vi "Test Get Objects in Range.vi"(11 "Test Case In":refnum<class "Test Object Dictionary.lvclass">) -> (0 "error out":errorcluster, 3 "Test Case Out":refnum<class "Test Object Dictionary.lvclass">)   [LabVIEW 2020, in "Test Object Dictionary.lvclass"]
uses:
  Test Object Dictionary.lvclass
  C:/Program Files/National Instruments/LabVIEW 2026/vi.lib/Astemes/LUnit/Test Case.lvclass
  EDS-File-Viewer/source/Electronic Datasheet/Electronic Datasheet.lvclass/Electronic Datasheet.ctl
  source/Object Entry/Object Entry.lvclass/Object Entry.ctl
  source/Sub Object/Sub Object.lvclass/Sub Object.ctl
  <vilib>/Astemes/LUnit/Test Case.lvclass/Test Case.ctl
  source/Sub Object/Sub Object.lvclass
  EDS-File-Viewer/source/Electronic Datasheet/Electronic Datasheet.lvclass
  source/Typedefs/Object Type.ctl
  source/CANopen.lvlib
  <vilib>/Astemes/LUnit/Test Case.lvclass
  source/Object Dictionary/Object Dictionary.lvclass
  source/Object Entry/Object Entry.lvclass
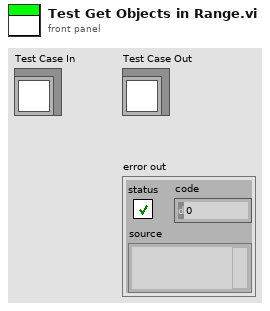
[diagram p1: front panel]
types:
  T1 = typedef "CANopen.lvlib/Object Type.ctl" = u8
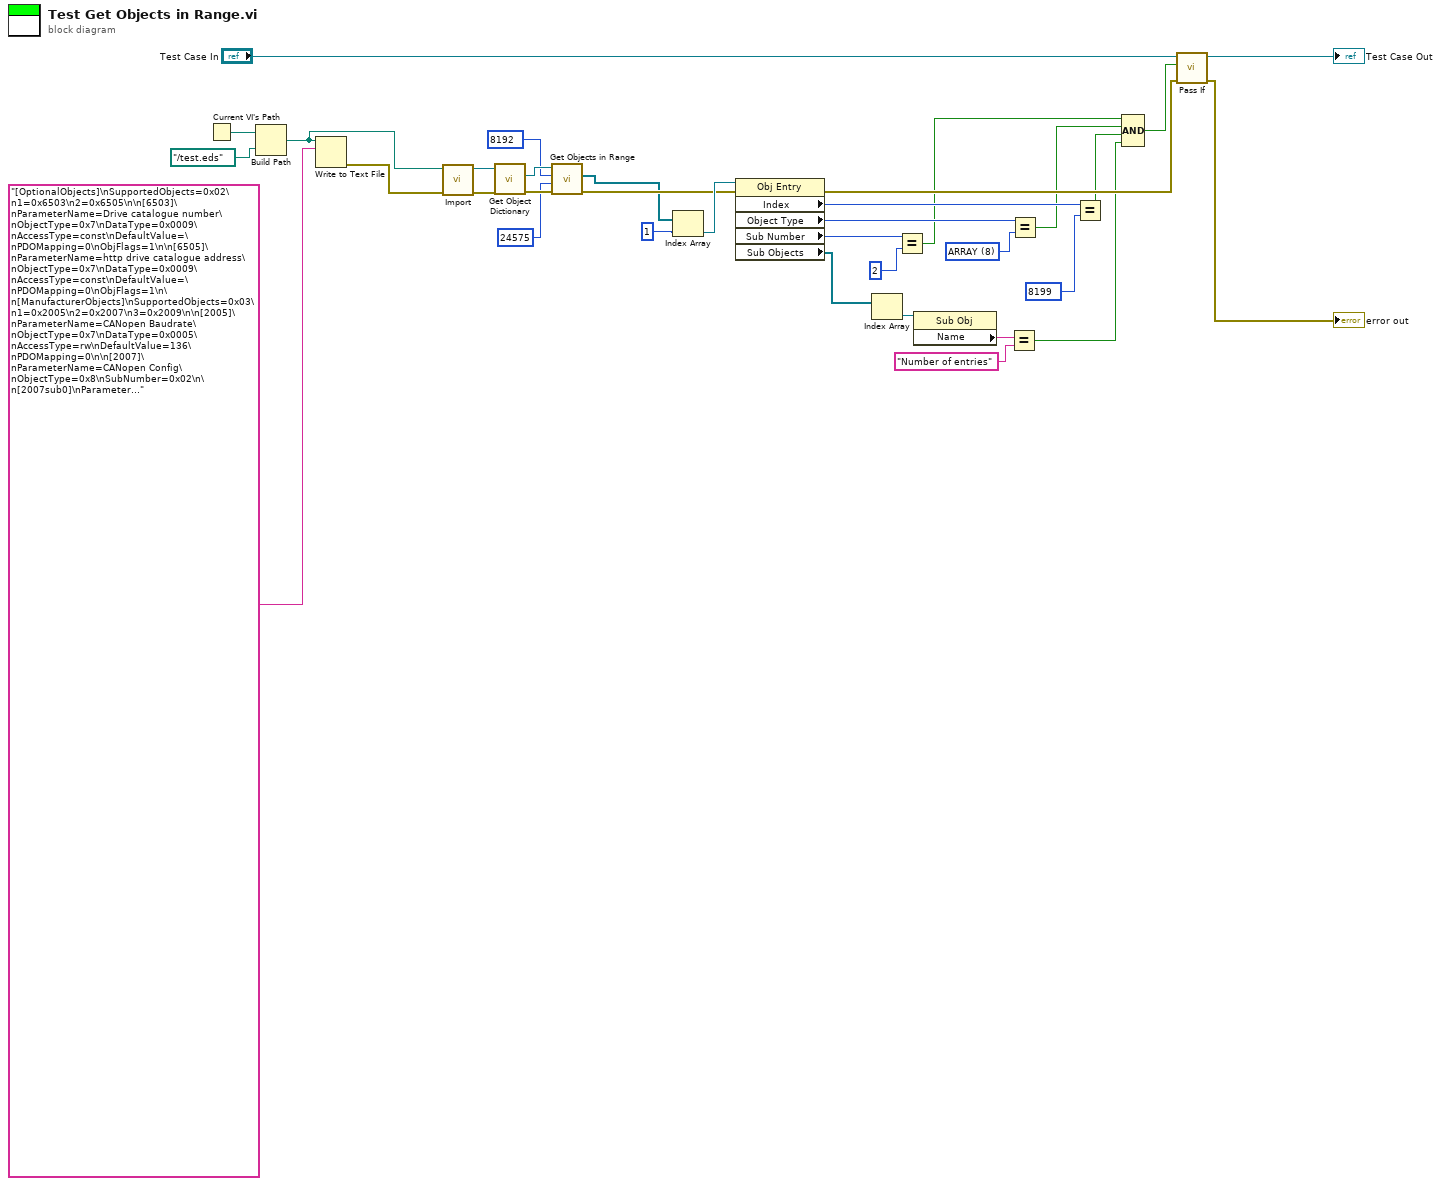
[diagram p0: block diagram]
diagram:
  w20 = T1 8 items=["NULL"=0, "DOMAIN"=2, "DEFTYPE"=5, "DEFSTRUCT"=6, "VAR"=7, "ARRAY"=8, "RECORD"=9] ("y")
  n1 = Current VI's Path() -> (path=w31:path)
  n2 = Build Path(base path=w31, name or relative path=path "../test.eds") -> (appended path=w29:path)
  n3 = Write to Text File(file (use dialog)=w29, text="[OptionalObjects]\nSupportedObjects=0x02\n1=0x6503\n2=0x6505\n\n[6503]\nParameterName=Drive catalogue number\nObjectType=0x7\nDataType=0x0009\nAccessType=const\nDefaultValue=\nPDOMapping=0\nObjFlags=1\n\n[6505]\nParameterName=http drive catalogue address\nObjectType=0x7\nDataType=0x0009\nAccessType=const\nDefaultValue=\nPDOMapping=0\nObjFlags=1\n\n[ManufacturerObjects]\nSupportedObjects=0x03\n1=0x2005\n2=0x2007\n3=0x2009\n\n[2005]\nParameterName=CANopen Baudrate\nObjectType=0x7\nDataType=0x0005\nAccessType=rw\nDefaultValue=136\nPDOMapping=0\n\n[2007]\nParameterName=CANopen Config\nObjectType=0x8\nSubNumber=0x02\n\n[2007sub0]\nParameterName=Number of entries\nObjectType=0x7\nDataType=0x0005\nAccessType=const\nDefaultValue=0x01\nPDOMapping=0\n\n[2007sub1]\nParameterName=BL Config\nObjectType=0x7\nDataType=0x0007\nAccessType=rw\nDefaultValue=0x00000000\nPDOMapping=0\n\n[2009]\nParameterName=CANopen NodeID\nObjectType=0x7\nDataType=0x0005\nAccessType=rw\nDefaultValue=0x7F\nPDOMapping=0\n") -> (error out=w28:errorcluster)  [unwired: 2 in, 2 out]
  n4 = call "Import.vi"("error in"=w28, "EDS File Path"=w29) -> ("error out"=w27:errorcluster, "Electronic Datasheet"=w26:refnum<class "Electronic Datasheet.lvclass">)  [unwired: 8 in]
  n5 = call "Get Object Dictionary.vi"("error in"=w27, "Electronic Datasheet in"=w26) -> ("error out"=w25:errorcluster, "Obj Dict"=w4:refnum<class "Object Dictionary.lvclass">)  [unwired: 7 in, 1 out]
  n6 = call "Get Objects in Range.vi"("error in"=w25, "End"=u16 24575, "Start"=u16 8192, "Obj Dict in"=w4) -> ("error out"=w5:errorcluster, "Objects in Range"=w1:refnum<class "Object Entry.lvclass">[])  [unwired: 5 in, 1 out]
  n7 = Index Array(array=w1, index=1) -> (element=w22:refnum<class "Object Entry.lvclass">)
  n8 = property class="Obj Entry"(reference=w22, error in=w5) -> (error out=w23:errorcluster, "Index"=w19:u16, "Object Type"=w21:T1, "Sub Number"=w17:u8, "Sub Objects"=w11:refnum<class "Sub Object.lvclass">[])  [unwired: 1 out]
  n9 = Index Array(array=w11) -> (element=w10:refnum<class "Sub Object.lvclass">)  [unwired: 1 in]
  n10 = Equal?(x=w17, y=u8 2) -> (x = y?=w15:bool)
  n11 = property class="Sub Obj"(reference=w10) -> ("Name"=w9:string)  [unwired: 1 in, 2 out]
  n12 = Equal?(x=w9, y="Number of entries") -> (x = y?=w7:bool)
  n13 = Equal?(x=w21, y=w20) -> (x = y?=w14:bool)
  n14 = Equal?(x=w19, y=u16 8199) -> (x = y?=w13:bool)
  n15 = Compound Arithmetic op=AND(w15, w14, w13, w7) -> (w12:bool)
  n16 = call <vilib>:"Pass If.vi"("error in (no error)"=w23, "Pass?"=w12, "LUnit Test Case In"="Test Case In") -> ("error out"=→"error out":errorcluster, "LUnit Test Case Out"=→"Test Case Out":refnum<class "Test Object Dictionary.lvclass">)  [unwired: 7 in]
